vi "MoveToPosition.vi"(10 "Y":i32, 11 "X":i32) -> ()   [LabVIEW 2020]
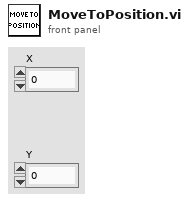
[diagram p1: front panel]
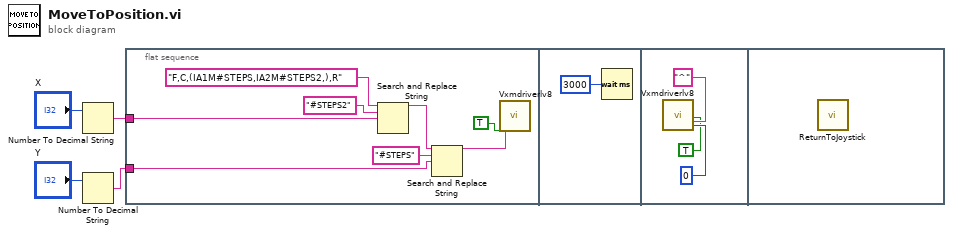
[diagram p0: block diagram]
diagram:
  n1 = Number To Decimal String(number="X") -> (decimal integer string=w4:string)  [unwired: 1 in]
  n2 = Number To Decimal String(number="Y") -> (decimal integer string=w3:string)  [unwired: 1 in]
  n3 = flat-sequence {
    tunnel: w3 -> [w6]
    tunnel: w4 -> [w5]
    frame #0 {
      n4 = Search and Replace String(input string="F,C,(IA1M#STEPS,IA2M#STEPS2,),R" ("Chars to send"), search string="#STEPS2", replace string=w5) -> (result string=w9:string)  [unwired: 5 in, 3 out]
      n5 = Search and Replace String(input string=w9, search string="#STEPS", replace string=w6) -> (result string=w10:string)  [unwired: 5 in, 3 out]
      n6 = call "Vxmdriverlv8.Vi"("Send\nchars\nto port"=TRUE, "Chars to send"=w10) -> ()  [unwired: 20 in, 6 out]
    }
    frame #1 {
      n7 = Wait (ms)(milliseconds to wait=u32 3000) -> ()  [unwired: 1 out]
    }
    frame #2 {
      n8 = call "Vxmdriverlv8.Vi"("Wait\nfor \nchar"=TRUE, "Char(s) to wait for"="^", "Char\nTimeout\nTime (ms)"=0) -> ()  [unwired: 19 in, 6 out]
    }
    frame #3 {
      n9 = call "ReturnToJoystick.vi"() -> ()  [unwired: 12 in]
    }
  }
